vi "Init Runtime.vi"(8 "error in (no error)":errorcluster, 10 "data allocations":T1, 11 "Wait On Boolean Step Config in":refnum<class "Wait On Boolean Step Config.lvclass">) -> (0 "error out":errorcluster, 2 "Skip":bool, 3 "Wait On Boolean Step Config out":refnum<class "Wait On Boolean Step Config.lvclass">)   [LabVIEW 2015, in "Wait On Boolean Step Config.lvclass"]
uses:
  Config/Wait On Boolean Step Config.lvclass
  <vilib>/NI/Tag Bus Module Framework/channel/data tables.ctl
  <vilib>/NI/Tag Bus/dictionary/data dictionary.lvclass
  <vilib>/NI/Tag Bus/dictionary table pair.ctl
  <vilib>/NI/Tag Bus/table/data table.ctl
  Wait On Boolean Step.lvclass
  classes/Step/Execution/StepState.ctl
  classes/Step/Execution/Step State Enum.ctl
  classes/Step/Execution/Step Flow Control.ctl
  <vilib>/NI/Tag Bus/tag/tag descriptor.lvclass/tag descriptor.ctl
  Wait On Boolean Step.lvclass/Wait On Boolean Step.ctl
  Write Channel Index.vi
  Write Timeout (ms).vi
  Write Pass.vi
  Write Timed Out.vi
  <vilib>/NI/Tag Bus/tag/read tag name.vi
  <vilib>/NI/Tag Bus/tag/read data type.vi
  <vilib>/NI/Tag Bus/dictionary/locate tag.vi
  <vilib>/NI/Tag Bus Module Framework/channel/TBM channel.lvclass
  classes/Step/Execution/Step.lvclass
  <vilib>/NI/Tag Bus/table/data table.lvlib
  <vilib>/NI/Tag Bus/tag bus.lvlib
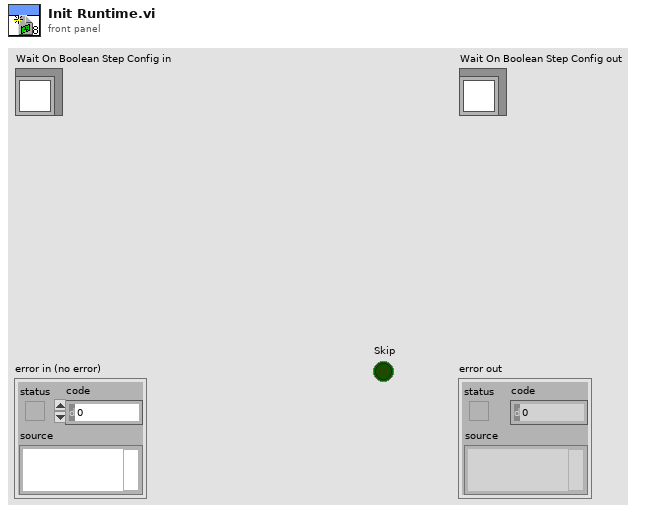
[diagram p1: front panel]
types:
  T1 = typedef "TBM channel.lvclass/data tables.ctl" = cluster{"input data":T2, "processing parameter":T2, "processing result":T2, "output data":T2}
  T2 = typedef "tag bus.lvlib/dictionary table pair.ctl" = cluster{"data dictionary":refnum<class "data dictionary.lvclass">, "data table":T3}
  T3 = typedef "tag bus.lvlib/data table.lvlib/data table.ctl" = cluster{"Double":dbl[], "Single":sgl[], "I64":i64[], "I32":i32[], "I16":i16[], "I8":i8[], "U64":u64[], "U32":u32[], "U16":u16[], "U8":u8[], "Boolean":bool[], "String":string[], "Array of Double":cluster{"DBL Array":dbl[]}[], "Array of Single":cluster{"SGL Array":sgl[]}[], "Array of I64":cluster{"I64 Array":i64[]}[], "Array of I32":cluster{"I32 Array":i32[]}[], "Array of I16":cluster{"I16 Array":i16[]}[], "Array of I8":cluster{"I8 Array":i8[]}[], "Array of U64":cluster{"U64 Array":u64[]}[], "Array of U32":cluster{"U32 Array":u32[]}[], "Array of U16":cluster{"U16 Array":u16[]}[], "Array of U8":cluster{"U8 Array":u8[]}[], "Array of Boolean":cluster{"Boolean Array":bool[]}[], "Array of String":cluster{"String Array":string[]}[]}
  T4 = typedef "Step.lvclass/StepState.ctl" = cluster{"Step State":T5, "Flow Control":T6, "Jump Index":i32}
  T5 = typedef "Step.lvclass/Step State Enum.ctl" = enum16{"Start", "Skipped", "Timeout", "Completed", "Running", "Aborted"}
  T6 = typedef "Step.lvclass/Step Flow Control.ctl" = enum16{"Next Step", "Jump"}
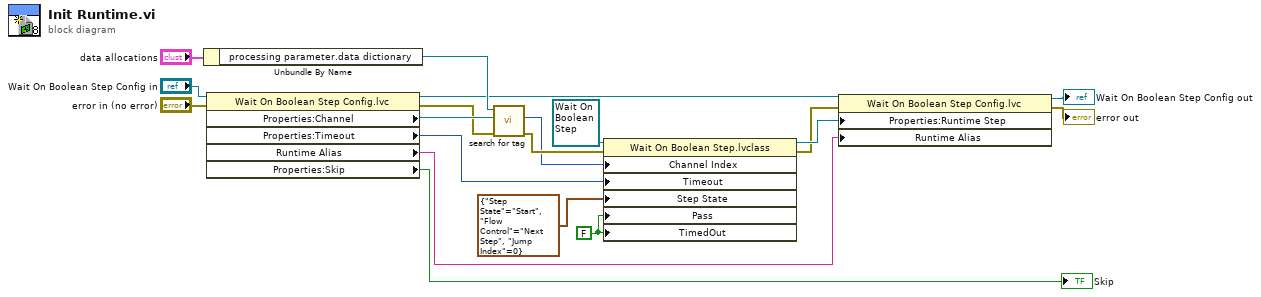
[diagram p0: block diagram]
diagram:
  w9 = FALSE ("Results")
  n1 = Unbundle By Name("data allocations") -> ("processing parameter.data dictionary"=w12:refnum<class "data dictionary.lvclass">)
  n2 = property class="Wait On Boolean Step Config.lvc"(reference="Wait On Boolean Step Config in", error in="error in (no error)") -> (reference out=w7:refnum<class "Wait On Boolean Step Config.lvclass">, error out=w4:errorcluster, "Properties:Channel"=w6:refnum<class "TBM channel.lvclass">, "Properties:Timeout"=w2:i32, "Runtime Alias"=w3:string, "Properties:Skip"=→"Skip":bool)
  n3 = call <vilib>:"search for tag.vi"("error in"=w4, "system tag"=w6, "data dictionary in"=w12) -> ("error out"=w10:errorcluster, "index"=w1:i32)  [unwired: 6 in, 1 out]
  n4 = property class="Wait On Boolean Step.lvclass"(reference=refnum<class "Wait On Boolean Step.lvclass"> refnum ("Wait On Boolean Step.lvclass"), error in=w10, "Channel Index"=w1, "Timeout"=w2, "Step State"=T4 {"Step State"=enum."Start", "Flow Control"=enum."Next Step", "Jump Index"=0}, "Pass"=w9, "TimedOut"=w9) -> (reference out=w17:refnum<class "Wait On Boolean Step.lvclass">, error out=w16:errorcluster)
  n5 = property class="Wait On Boolean Step Config.lvc"(reference=w7, error in=w16, "Properties:Runtime Step"=w17, "Runtime Alias"=w3) -> (reference out=→"Wait On Boolean Step Config out":refnum<class "Wait On Boolean Step Config.lvclass">, error out=→"error out":errorcluster)
